vi "BPM-Chassis02 FPGA.vi"() -> ()   [LabVIEW 2010]
uses:
  <vilib>/eio/EIONode/EIONode.xnode
  <vilib>/rvi/eio/nirviEIOImplementation/nirviEIOImplementation.xnode
  <vilib>/rvi/eio/common/nirviEmuClasses.ctl
  <vilib>/eio/EIOMethodNode/EIOMethodNode.xnode
  <vilib>/rvi/eio/nirviEIOMethodImplementation/nirviEIOMethodImplementation.xnode
  <vilib>/rvi/Analysis/measure/butterworth/XNode/niFpgaButterworthFilter.xnode
  <vilib>/rvi/eio/common/nirviEmuTemplateMethod_noerrors.vi
panel:
  out "Mod1/AI1":fxp<+/-,20,5> format="%.17g"
  out "Mod2/AI3":fxp<+/-,20,5> format="%.17g"
  out "Mod2/AI2":fxp<+/-,20,5> format="%.17g"
  out "Mod2/AI1":fxp<+/-,20,5> format="%.17g"
  out "Mod2/AI0":fxp<+/-,20,5> format="%.17g"
  out "Mod1/AI3":fxp<+/-,20,5> format="%.17g"
  out "Mod1/AI2":fxp<+/-,20,5> format="%.17g"
  out "Mod1/AI0":fxp<+/-,20,5> format="%.17g"
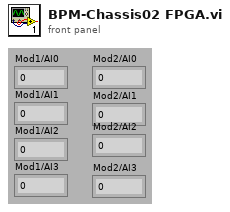
[diagram p1: front panel]
types:
  T1 = typedef "nirviEmuClasses.ctl" = enum16{"IO Read", "IO Write", "Method", "Property Read", "Property Write"}
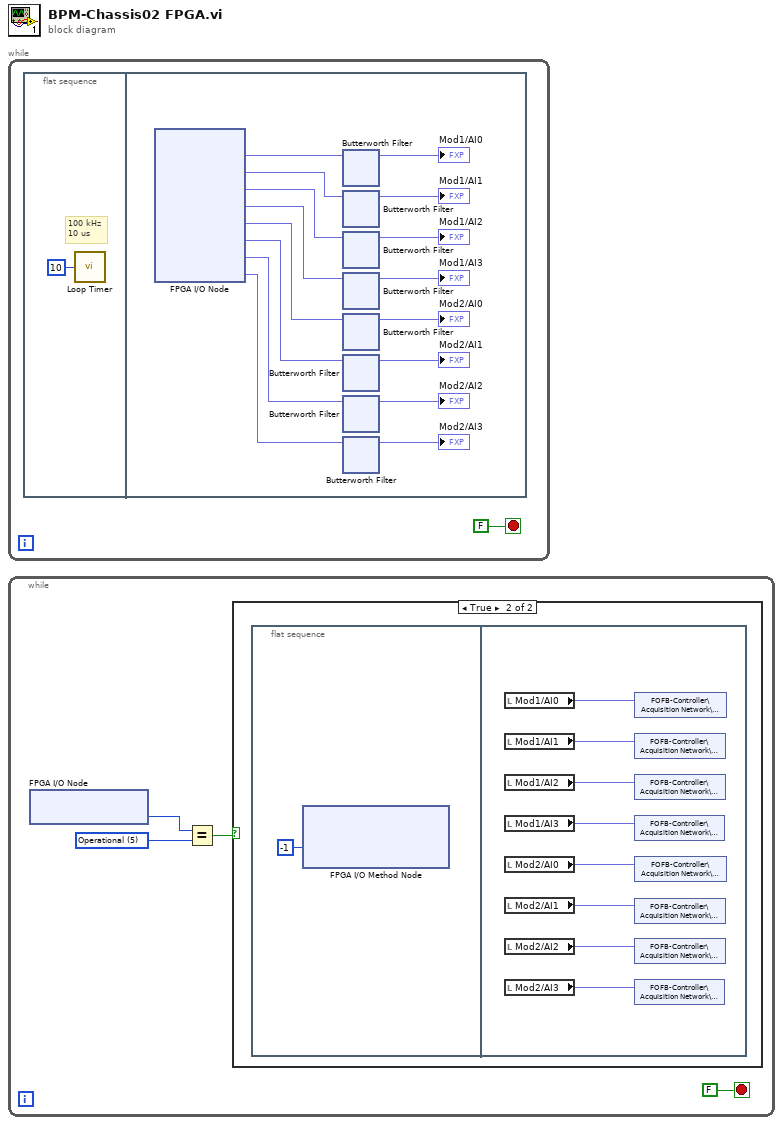
[diagram p0: block diagram]
diagram:
  n1 = while {
    stop <- FALSE stop-if-true
    n2 = flat-sequence {
      frame #0 {
        # "100 kHz\n10 us"
        n3 = call "Loop Timer"("Count(uSec)"=u8 10) -> ()  [unwired: 1 out]
      }
      frame #1 {
        n4 = xnode "FPGA I/O Node"() -> ("Mod1/AI0"=w18:fxp<+/-,20,5>, "Mod1/AI1"=w14:fxp<+/-,20,5>, "Mod1/AI2"=w13:fxp<+/-,20,5>, "Mod1/AI3"=w12:fxp<+/-,20,5>, "Mod2/AI0"=w11:fxp<+/-,20,5>, "Mod2/AI1"=w10:fxp<+/-,20,5>, "Mod2/AI2"=w9:fxp<+/-,20,5>, "Mod2/AI3"=w16:fxp<+/-,20,5>)  [unwired: 8 in, 8 out]
        n5 = xnode "Butterworth Filter"("input data"=w18) -> ("output data"=→"Mod1/AI0":fxp<+/-,20,5>)  [unwired: 2 in]
        n6 = xnode "Butterworth Filter"("input data"=w14) -> ("output data"=→"Mod1/AI1":fxp<+/-,20,5>)  [unwired: 2 in]
        n7 = xnode "Butterworth Filter"("input data"=w13) -> ("output data"=→"Mod1/AI2":fxp<+/-,20,5>)  [unwired: 2 in]
        n8 = xnode "Butterworth Filter"("input data"=w12) -> ("output data"=→"Mod1/AI3":fxp<+/-,20,5>)  [unwired: 2 in]
        n9 = xnode "Butterworth Filter"("input data"=w11) -> ("output data"=→"Mod2/AI0":fxp<+/-,20,5>)  [unwired: 2 in]
        n10 = xnode "Butterworth Filter"("input data"=w10) -> ("output data"=→"Mod2/AI1":fxp<+/-,20,5>)  [unwired: 2 in]
        n11 = xnode "Butterworth Filter"("input data"=w9) -> ("output data"=→"Mod2/AI2":fxp<+/-,20,5>)  [unwired: 2 in]
        n12 = xnode "Butterworth Filter"("input data"=w16) -> ("output data"=→"Mod2/AI3":fxp<+/-,20,5>)  [unwired: 2 in]
      }
    }
  }
  n13 = while {
    stop <- FALSE stop-if-true
    w245 = u8 5 items=["Init"=1, "PreOp"=2, "Bootstrap"=3, "SafeOp"=4, "Operational"=5]
    n14 = xnode "FPGA I/O Node"() -> ("EtherCAT State"=w244:u8)  [unwired: 1 in, 1 out]
    n15 = Equal?(x=w244, y=w245) -> (x = y?=w243:bool)
    n16 = case shown="True" w243 {
      frame False {
      }
      frame True {
        n17 = flat-sequence {
          frame #0 {
            n18 = xnode "FPGA I/O Method Node"("Timeout"=-1) -> ()  [unwired: 1 in, 2 out]
          }
          frame #1 {
            n19 = local read "Mod1/AI0"() -> (w278:fxp<+/-,20,5>)
            n20 = local read "Mod1/AI1"() -> (w276:fxp<+/-,20,5>)
            n21 = local read "Mod1/AI2"() -> (w275:fxp<+/-,20,5>)
            n22 = local read "Mod1/AI3"() -> (w274:fxp<+/-,20,5>)
            n23 = local read "Mod2/AI0"() -> (w273:fxp<+/-,20,5>)
            n24 = local read "Mod2/AI1"() -> (w272:fxp<+/-,20,5>)
            n25 = local read "Mod2/AI2"() -> (w271:fxp<+/-,20,5>)
            n26 = local read "Mod2/AI3"() -> (w277:fxp<+/-,20,5>)
            n27 = shared-variable "FOFB-Controller\\Acquisition Network\\BPM-Chassis02\\User-Defined Variables\\AMP04AH"(w278) -> ()  [unwired: 1 in, 1 out]
            n28 = shared-variable "FOFB-Controller\\Acquisition Network\\BPM-Chassis02\\User-Defined Variables\\AMP04AV"(w276) -> ()  [unwired: 1 in, 1 out]
            n29 = shared-variable "FOFB-Controller\\Acquisition Network\\BPM-Chassis02\\User-Defined Variables\\AMP04BH"(w275) -> ()  [unwired: 1 in, 1 out]
            n30 = shared-variable "FOFB-Controller\\Acquisition Network\\BPM-Chassis02\\User-Defined Variables\\AMP04BV"(w274) -> ()  [unwired: 1 in, 1 out]
            n31 = shared-variable "FOFB-Controller\\Acquisition Network\\BPM-Chassis02\\User-Defined Variables\\AMP05AH"(w273) -> ()  [unwired: 1 in, 1 out]
            n32 = shared-variable "FOFB-Controller\\Acquisition Network\\BPM-Chassis02\\User-Defined Variables\\AMP05AV"(w272) -> ()  [unwired: 1 in, 1 out]
            n33 = shared-variable "FOFB-Controller\\Acquisition Network\\BPM-Chassis02\\User-Defined Variables\\AMP05BH"(w271) -> ()  [unwired: 1 in, 1 out]
            n34 = shared-variable "FOFB-Controller\\Acquisition Network\\BPM-Chassis02\\User-Defined Variables\\AMP05BV"(w277) -> ()  [unwired: 1 in, 1 out]
          }
        }
      }
    }
  }
